vi "Write Coordinates.CAD Cluster.vi"(8 "error in (no error)":errorcluster, 10 "Coordinates.CAD Cluster":T1(array[cluster]), 11 "Sensor Dispense in":refnum<class "Sensor Dispense.lvclass">) -> (0 "error out":errorcluster, 3 "Sensor Dispense out":refnum<class "Sensor Dispense.lvclass">)   [LabVIEW 2018, in "Sensor Dispense.lvclass"]
uses:
  Projects/Sensor Dispense.lvclass
  Projects/Sensor Dispense.lvclass/Sensor Dispense.ctl
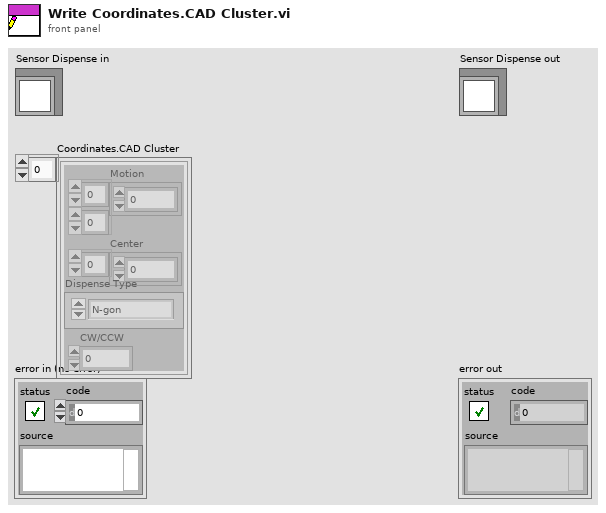
[diagram p1: front panel]
types:
  T1 = cluster{"Motion":dbl[][], "Center":dbl[], "CW/CCW":dbl, "Dispense Type":enum16{"N-gon", "Square", "Arc", "Dot", "Line", "Circle"}}[]
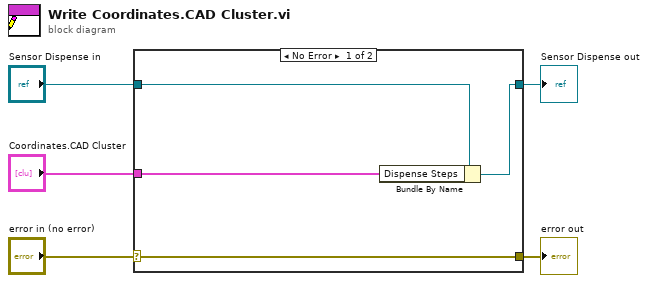
[diagram p0: block diagram]
diagram:
  n1 = case shown="No Error" "error in (no error)" {
    selector: "error in (no error)" -> [w9 w10]
    tunnel: [w9 w10] -> w4
    tunnel: [w7 w11] -> w2
    tunnel: "Sensor Dispense in" -> [w8 w11]
    tunnel: "Coordinates.CAD Cluster" -> [w6 _]
    frame No Error {
      n2 = Bundle By Name(cluster=w8, "Dispense Steps"=w6) -> (w7:refnum<class "Sensor Dispense.lvclass">)
    }
    frame Error {
    }
  }
  "error out" <- w4
  "Sensor Dispense out" <- w2
